vi "Begin.vi"(8 "error in":errorcluster) -> (0 "error out":errorcluster)   [LabVIEW 2020]
doc: "Called before other user functions, this VI is expected to open initial I/O refnums, load in file data, and do all program initialization. Notice that the <B>error out</B> terminal is simply used for data flow. Wiring it to other structures or subVIs ensures that this VI runs first."
uses:
  <vilib>/Rock Robotics/WPI/DriverStation/WPI_DriverStationRobotMode2.ctl
  <vilib>/Rock Robotics/WPI/Joystick/WPI_JoystickDeviceEnum.ctl
  <vilib>/Rock Robotics/SystemInterfaces/DIO/FPGA_DIOChannel.ctl
  Robot Global Data.vi
  <vilib>/Rock Robotics/Network Tables/NT Write String Array.vi
  <vilib>/Rock Robotics/WPI/Solenoid/WPI_SolenoidOpenDouble.vi
  <vilib>/Rock Robotics/WPI/Solenoid/WPI_SolenoidChannel.ctl
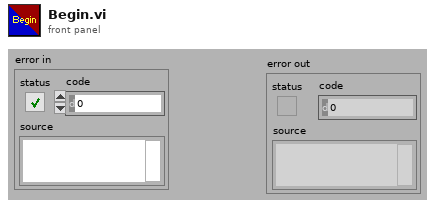
[diagram p1: front panel]
types:
  T1 = typedef "WPI_SolenoidChannel.ctl" = enum8{"Solenoid 0", "Solenoid 1", "Solenoid 2", "Solenoid 3", "Solenoid 4", "Solenoid 5", "Solenoid 6", "Solenoid 7", "Solenoid 8", "Solenoid 9", "Solenoid 10", "Solenoid 11", "Solenoid 12", "Solenoid 13", "Solenoid 14", "Solenoid 15", "Invalid"}
  T2 = typedef "FPGA_DIOChannel.ctl" = enum8{"DIO 0", "DIO 1", "DIO 2", "DIO 3", "DIO 4", "DIO 5", "DIO 6", "DIO 7", "DIO 8", "DIO 9", "DIO MXP 0", "DIO MXP 1", "DIO MXP 2", "DIO MXP 3", "DIO MXP 4", "DIO MXP 5", "DIO MXP 6", "DIO MXP 7", "DIO MXP 8", "DIO MXP 9", "DIO MXP 10", "DIO MXP 11", "DIO MXP 12", "DIO MXP 13", "DIO MXP 14", "DIO MXP 15", "SPI Port CS1", "SPI Port CS2", "SPI Port CS3", "SPI Port MISO", "SPI Port MOSI", "Invalid"}
  T3 = typedef "WPI_JoystickDeviceEnum.ctl" = enum16{"USB 0", "USB 1", "USB 2", "USB 3", "USB 4", "USB 5"}
  T4 = typedef "WPI_DriverStationRobotMode2.ctl" = enum16{"Autonomous Disabled", "Autonomous Enabled", "Teleop Disabled", "Teleop Enabled", "Disconnected", "Finish", "Test Disabled", "Test Enabled", "Emergency Stopped"}
  T5 = typedef "WPI_JoystickDevRef.ctl" = cluster{"Device":T3}
  T6 = typedef "WPI_MotorControlDeviceRef.ctl" = cluster{"DeviceStatus":errorcluster, "Type":T7, "PWM":cluster{"PWM Channel":T8, "DeadBand":T9}, "CAN":cluster{"Device Number":u8, "SetOutput VI Ref":variant, "GetOutput VI Ref":variant, "Enable VI Ref":variant, "Disable VI Ref":variant, "Data":variant}, "Invert":bool, "DIO PWM":cluster{"PWM \"Enable\" Channel":T8, "DIOChannel":T2, "PWM Rate":dbl}}
  T7 = typedef "WPI_MotorControlType.ctl" = enum16{"PWM", "CAN", "DIO PWM"}
  T8 = typedef "FPGA_DIOPWMChannel.ctl" = enum8{"PWM 0", "PWM 1", "PWM 2", "PWM 3", "PWM 4", "PWM 5", "PWM 6", "PWM 7", "PWM 8", "PWM 9", "PWM MXP 0", "PWM MXP 1", "PWM MXP 2", "PWM MXP 3", "PWM MXP 4", "PWM MXP 5", "PWM MXP 6", "PWM MXP 7", "PWM MXP 8", "PWM MXP 9", "Invalid"}
  T9 = typedef "WPI_PWMDeadband.ctl" = cluster{"Name":string, "maxPositivePwm":i32, "minPositivePwm":i32, "centerPwm":i32, "maxNegativePwm":i32, "minNegativePwm":i32, "angularRange":u16}
  T10 = typedef "WPI_SolenoidDevRef.ctl" = cluster{"DevStatus":errorcluster, "Pneumatics Control Module":u8, "Forward Solenoid Channel":T1, "Reverse Solenoid Channel":T1}
  T11 = typedef "WPI_DigitalInputDevRef.ctl" = cluster{"DevStatus":errorcluster, "DIO Channel":T2}
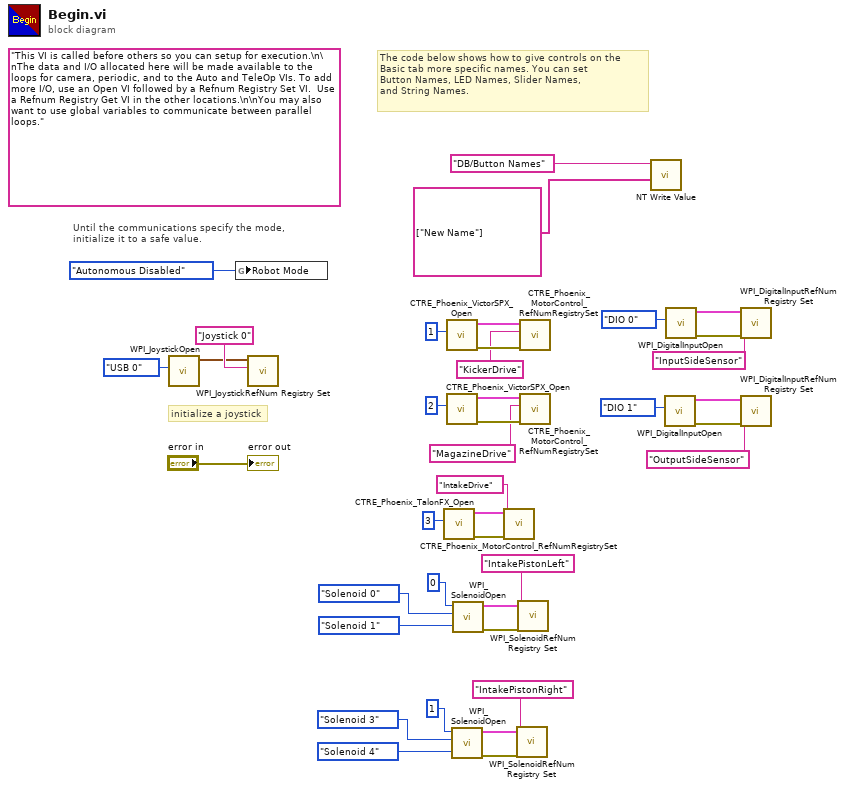
[diagram p0: block diagram]
diagram:
  (unwired) "This VI is called before others so you can setup for execution.\n\nThe data and I/O allocated here will be made available to the loops for camera, periodic, and to the Auto and TeleOp VIs. To add more I/O, use an Open VI followed by a Refnum Registry Set VI.  Use a Refnum Registry Get VI in the other locations.\n\nYou may also want to use global variables to communicate between parallel loops."
  # "The code below shows how to give controls on the\nBasic tab more specific names. You can set\nButton Names, LED Names, Slider Names,\nand String Names."
  # "initialize a joystick"
  # "Until the communications specify the mode,\ninitialize it to a safe value."
  n1 = call <vilib>:"WPI_JoystickOpen.vi"("JoystickDevice"=WPI_JoystickDeviceEnum."USB 0") -> ("JoystickDevRef"=w37:T5)  [unwired: 10 in]
  n2 = global write "Robot Global Data.vi" "Robot Mode"(WPI_DriverStationRobotMode2."Autonomous Disabled" ("Robot Mode")) -> ()
  n3 = call <vilib>:"WPI_JoystickRefNum Registry Set.vi"("refnum name"="Joystick 0", "JoystickDevRef"=w37) -> ()  [unwired: 8 in, 2 out]
  n4 = call <vilib>:"CTRE_Phoenix_TalonFX_Open.vi"("Device Number"=u8 3) -> ("error out"=w16:errorcluster, "PhoenixMotorControlDevRef"=w15:T6)  [unwired: 9 in]
  n5 = call <vilib>:"CTRE_Phoenix_VictorSPX_Open.vi"("Device Number"=u8 1) -> ("error out"=w32:errorcluster, "PhoenixMotorControlDevRef"=w31:T6)  [unwired: 9 in]
  n6 = call <vilib>:"CTRE_Phoenix_VictorSPX_Open.vi"("Device Number"=u8 2) -> ("error out"=w30:errorcluster, "PhoenixMotorControlDevRef"=w29:T6)  [unwired: 9 in]
  n7 = call-poly <vilib>:"WPI_SolenoidOpen.vi"("Reverse Solenoid Channel"=WPI_SolenoidChannel."Solenoid 4", "Forward Solenoid Channel"=WPI_SolenoidChannel."Solenoid 3", "Pneumatics Device (def)"=u8 1) -> ("error out"=w3:errorcluster, "SolenoidDevRef"=w2:T10)  [unwired: 7 in]
  n8 = call-poly <vilib>:"WPI_SolenoidOpen.vi"("Reverse Solenoid Channel"=WPI_SolenoidChannel."Solenoid 1", "Forward Solenoid Channel"=WPI_SolenoidChannel."Solenoid 0", "Pneumatics Device (def)"=u8 0) -> ("error out"=w9:errorcluster, "SolenoidDevRef"=w8:T10)  [unwired: 7 in]
  n9 = call <vilib>:"CTRE_Phoenix_MotorControl_RefNumRegistrySet.vi"("error in (no error)"=w16, "refnum name"="IntakeDrive", "PhoenixMotorControlDevRef"=w15) -> ()  [unwired: 7 in, 2 out]
  n10 = call <vilib>:"WPI_SolenoidRefNum Registry Set.vi"("error in (no error)"=w3, "refnum name"="IntakePistonRight", "SolenoidDevRef"=w2) -> ()  [unwired: 7 in, 2 out]
  n11 = call <vilib>:"WPI_SolenoidRefNum Registry Set.vi"("error in (no error)"=w9, "refnum name"="IntakePistonLeft", "SolenoidDevRef"=w8) -> ()  [unwired: 7 in, 2 out]
  n12 = call <vilib>:"CTRE_Phoenix_MotorControl_RefNumRegistrySet.vi"("error in (no error)"=w32, "refnum name"="KickerDrive", "PhoenixMotorControlDevRef"=w31) -> ()  [unwired: 7 in, 2 out]
  n13 = call <vilib>:"CTRE_Phoenix_MotorControl_RefNumRegistrySet.vi"("error in (no error)"=w30, "refnum name"="MagazineDrive", "PhoenixMotorControlDevRef"=w29) -> ()  [unwired: 7 in, 2 out]
  n14 = call-poly <vilib>:"NT Write Value.vi"("String Array"=string[] ["New Name"], "Name"="DB/Button Names") -> ()  [unwired: 9 in, 1 out]
  n15 = call <vilib>:"WPI_DigitalInputOpen.vi"("DIO Channel"=FPGA_DIOChannel."DIO 1") -> ("error out"=w24:errorcluster, "DigitalInputDevRef"=w23:T11)  [unwired: 9 in]
  n16 = call <vilib>:"WPI_DigitalInputOpen.vi"("DIO Channel"=FPGA_DIOChannel."DIO 0") -> ("error out"=w22:errorcluster, "DigitalInputDevRef"=w21:T11)  [unwired: 9 in]
  n17 = call <vilib>:"WPI_DigitalInputRefNum Registry Set.vi"("error in (no error)"=w22, "refnum name"="InputSideSensor", "DigitalInputDevRef"=w21) -> ()  [unwired: 7 in, 2 out]
  n18 = call <vilib>:"WPI_DigitalInputRefNum Registry Set.vi"("error in (no error)"=w24, "refnum name"="OutputSideSensor", "DigitalInputDevRef"=w23) -> ()  [unwired: 7 in, 2 out]
  "error out" <- "error in"
